vi "Visa Read All.vi"(8 "error in (no error)":errorcluster, 10 "Byte Count Each Loop (6000)":i32=6000, 11 "VISA resource name":refnum<visa-resource-name>) -> (0 "error out":errorcluster, 2 "Read Buffer":string, 3 "VISA resource name out":refnum<visa-resource-name>)   [LabVIEW 2023, in "Agilent B2900 Series.lvlib"]
doc: "Fetch the visa read buffer recursively until it is empty."
uses:
  Agilent B2900 Series.lvlib
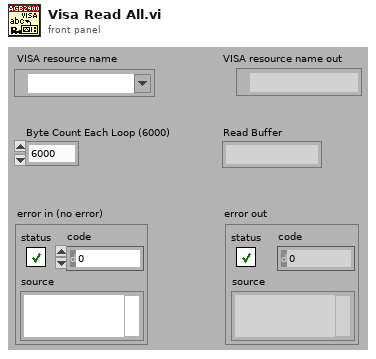
[diagram p1: front panel]
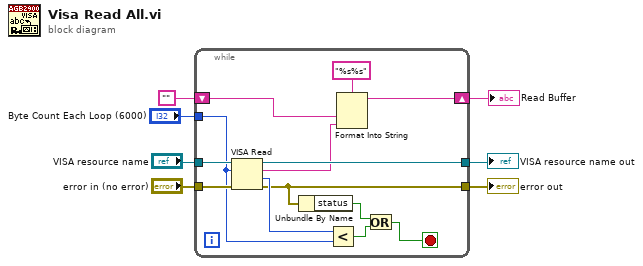
[diagram p0: block diagram]
diagram:
  n1 = while {
    tunnel: "VISA resource name" -> [w20]
    tunnel: "error in (no error)" -> [w19]
    tunnel: [w18] -> w5
    tunnel: [w15] -> w4
    tunnel: "Byte Count Each Loop (6000)" -> [w16]
    shift-right: [w8] -> w2
    shift-left: "" -> [w10]
    stop <- w12 stop-if-true
    n2 = VISA Read(VISA resource name=w20, byte count=w16, error in (no error)=w19) -> (VISA resource name out=w18:refnum<visa-resource-name>, read buffer=w9:string, return count=w17:u32, error out=w15:errorcluster)
    n3 = Unbundle By Name(w15) -> ("status"=w14:bool)
    n4 = Less?(x=w17, y=w16) -> (x < y?=w13:bool)
    n5 = Format Into String(format string="%s%s", w10, w9) -> (resulting string=w8:string)  [unwired: 2 in, 1 out]
    n6 = Or(x=w14, y=w13) -> (x .or. y?=w12:bool)
  }
  "VISA resource name out" <- w5
  "error out" <- w4
  "Read Buffer" <- w2
